vi "deney_8.1.2.vi"() -> ()   [LabVIEW 2018]
panel:
  out "Önceki Tahmin":dbl
  out "SAYI":u16
  in  "Tahmin":u16
  out "BITTI":bool
  out "KALAN":i32=10
  out "MESAJ":string="Tahmin : 0 .. 1023"
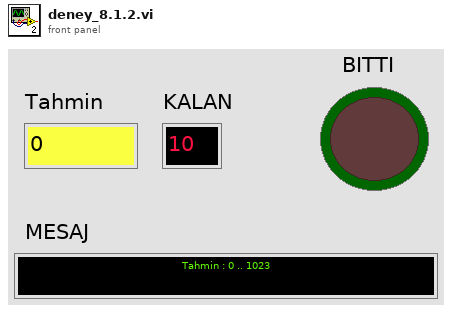
[diagram p1: front panel]
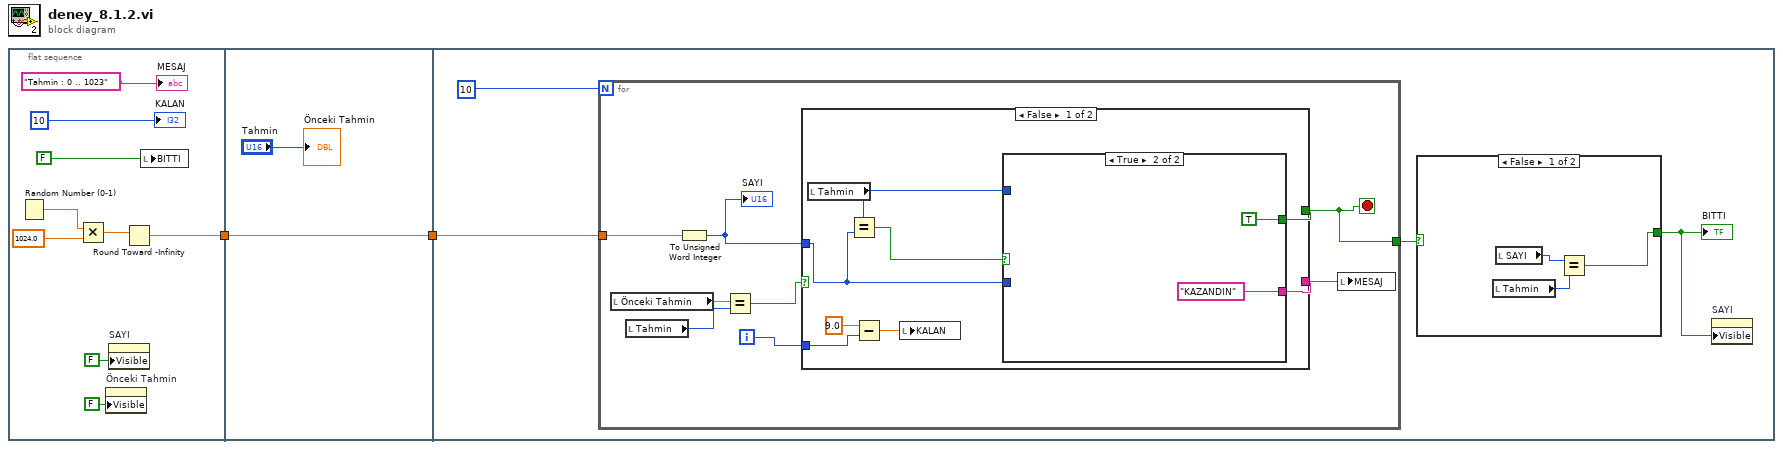
[diagram p0: block diagram]
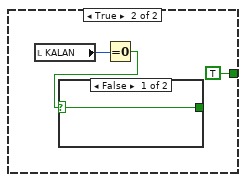
[diagram p2: hidden frame]
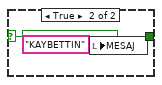
[diagram p3: hidden frame]
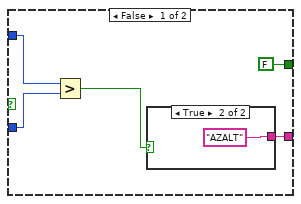
[diagram p4: hidden frame]
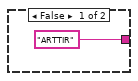
[diagram p5: hidden frame]
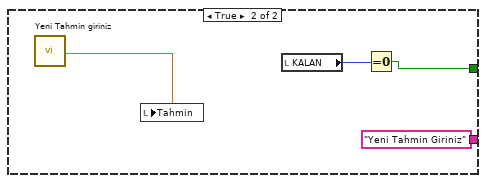
[diagram p6: hidden frame]
diagram:
  n1 = flat-sequence {
    tunnel: [w6] -> w2
    tunnel: w2 -> [w13]
    tunnel: [w13] -> w1
    tunnel: w1 -> [w16]
    frame #0 {
      n2 = Random Number (0-1)() -> (number: 0 to 1=w8:dbl)
      n3 = Multiply(x=w8, y=1024.0) -> (x*y=w7:dbl)
      n4 = property on="Önceki Tahmin" class="DigNum (strict)"("Visible"=FALSE) -> ()  [unwired: 2 in, 2 out]
      n5 = property on="SAYI" class="DigNum (strict)"("Visible"=FALSE) -> ()  [unwired: 2 in, 2 out]
      n6 = Round Toward -Infinity(1:w7) -> (0:w6:dbl)
      n7 = local write "BITTI"(FALSE ("BITTI")) -> ()
      "MESAJ" <- "Tahmin : 0 .. 1023"
      "KALAN" <- 10
    }
    frame #1 {
      "Önceki Tahmin" <- "Tahmin"
    }
    frame #2 {
      n8 = for {
        N: 10 -> [_]
        tunnel: w16 -> [w34]
        tunnel: [w27] -> w15
        i -> [w32]
        stop <- w27 stop-if-true
        n9 = local read "Önceki Tahmin"() -> (w30:dbl)
        n10 = local read "Tahmin"() -> (w29:u16)
        n11 = To Unsigned Word Integer(number=w34) -> (unsigned 16bit integer=w33:u16)
        "SAYI" <- w33
        n12 = Equal?(x=w30, y=w29) -> (x = y?=w28:bool)
        n13 = case shown="False" w28 {
          tunnel: w33 -> [w42 _]
          tunnel: w32 -> [w41 _]
          tunnel: [w40 "Yeni Tahmin Giriniz" ("MESAJ")] -> w31
          tunnel: [w39 w53] -> w27
          frame False {
            n14 = local read "Tahmin"() -> (w35:u16)
            n15 = Equal?(x=w35, y=w42) -> (x = y?=w38:bool)
            n16 = Subtract(x=9.0, y=w41) -> (x-y=w36:dbl)
            n17 = local write "KALAN"(w36) -> ()
            n18 = case shown="True" w38 {
              tunnel: w42 -> [w46 _]
              tunnel: w35 -> [w47 _]
              tunnel: [FALSE TRUE] -> w39
              tunnel: [w44 "KAZANDIN" ("MESAJ")] -> w40
              frame False {
                n19 = Greater?(x=w47, y=w46) -> (0:w45:bool)
                n20 = case shown="True" w45 {
                  tunnel: ["ARTTIR" ("MESAJ") "AZALT" ("MESAJ")] -> w44
                  frame False {
                  }
                  frame True {
                  }
                }
              }
              frame True {
              }
            }
          }
          frame True {
            n21 = call "Yeni Tahmin giriniz"() -> ("Tahmin"=w52:dbl)  [unwired: 17 in, 2 out]
            n22 = local write "Tahmin"(w52) -> ()
            n23 = local read "KALAN"() -> (w54:i32)
            n24 = Equal To 0?(x=w54) -> (x = 0?=w53:bool)
          }
        }
        n25 = local write "MESAJ"(w31) -> ()
      }
      n26 = case shown="False" w15 {
        tunnel: [w18 TRUE] -> w14
        frame False {
          n27 = local read "Tahmin"() -> (w19:u16)
          n28 = local read "SAYI"() -> (w20:u16)
          n29 = Equal?(x=w20, y=w19) -> (x = y?=w18:bool)
        }
        frame True {
          n30 = local read "KALAN"() -> (w22:i32)
          n31 = Equal To 0?(x=w22) -> (x = 0?=w21:bool)
          n32 = case shown="False" w21 {
            selector: w21 -> [w24 w25]
            tunnel: [w24 w25] -> _
            frame False {
            }
            frame True {
              n33 = local write "MESAJ"("KAYBETTIN" ("MESAJ")) -> ()
            }
          }
        }
      }
      "BITTI" <- w14
      n34 = property on="SAYI" class="DigNum (strict)"("Visible"=w14) -> ()  [unwired: 2 in, 2 out]
    }
  }
